vi "Read Edge Actors.vi"(11 "Base Root Actors in":refnum<class "Base Root Actors.lvclass">) -> (2 "Edge Actors":refnum<class "Actor.lvclass">[](array[class]))   [LabVIEW 2020, in "jettl.lvlib" / "Base Root Actors.lvlib" / "Base Root Actors.lvclass"]
uses:
  Base Root Actors.lvclass
  Actor/Actor.lvclass
  Base Root Actors.lvclass/Base Root Actors.ctl
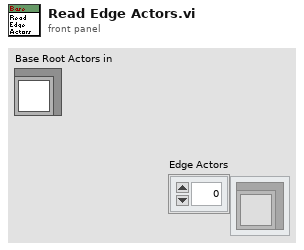
[diagram p1: front panel]
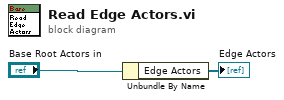
[diagram p0: block diagram]
diagram:
  n1 = Unbundle By Name("Base Root Actors in") -> ("Edge Actors"=→"Edge Actors":refnum<class "Actor.lvclass">[])
